vi "Single Waveform.vi"(8 "error in (no error)":errorcluster, 11 "Single Waveform":waveform(dbl)) -> (0 "error out":errorcluster, 2 "2D Array":dbl[][](array[numeric]))   [LabVIEW 2016]
doc: "This instance will convert a single waveform to a 2D array of doubles. The first column of the resulting 2D array will be the time data, indexed at 0."
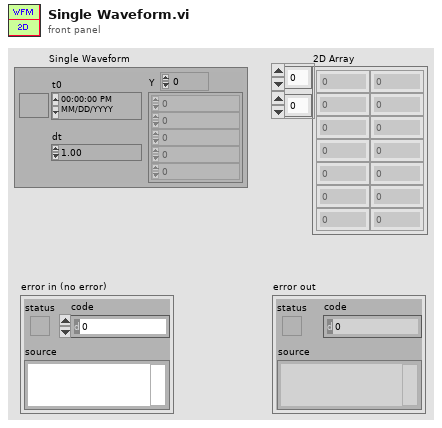
[diagram p1: front panel]
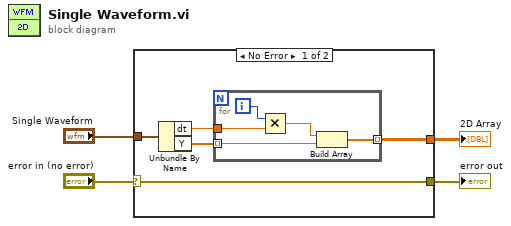
[diagram p0: block diagram]
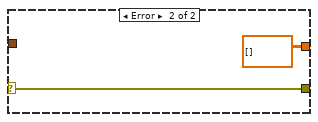
[diagram p2: hidden frame]
diagram:
  n1 = case shown="No Error" "error in (no error)" {
    selector: "error in (no error)" -> [w5 w16]
    tunnel: [w7 dbl[][] []] -> w4
    tunnel: "Single Waveform" -> [w6 _]
    tunnel: [w5 w16] -> w1
    frame No Error {
      n2 = Unbundle By Name(w6) -> ("dt"=w9:dbl, "Y"=w8:dbl[])
      n3 = for {
        tunnel: w9 -> [w14]
        tunnel: w8 -> [w12] mode=indexing
        tunnel: [w10] -> w7 mode=indexing
        i -> [w13]
        n4 = Multiply(x=w13, y=w14) -> (x*y=w11:dbl)
        n5 = Build Array(w11, w12) -> (w10:dbl[])
      }
    }
    frame Error {
    }
  }
  "2D Array" <- w4
  "error out" <- w1
